vi "Progress bar DAC scan.vi"(1 "Voltage (V)":dbl format="%.3f", 2 "DAC code":u16) -> (0 "Abort":bool, 3 "Prog Bar Ref":refnum<vi>)   [LabVIEW 2015]
panel:
  in  "Abort":bool
  out "DAC code":u16(slide) scale=0.0..65535.0
  # "DAC Scan Progress"
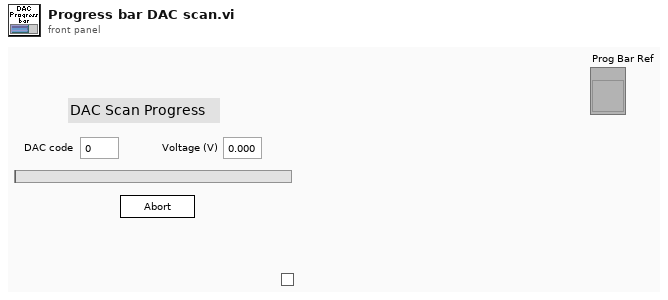
[diagram p1: front panel]
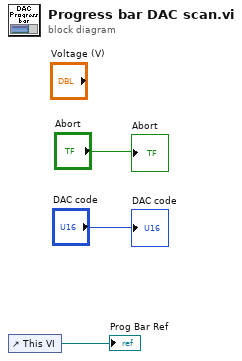
[diagram p0: block diagram]
diagram:
  n1 = control-ref of="This VI"() -> (→"Prog Bar Ref":refnum<vi>)
  "DAC code" <- "DAC code"
  "Abort" <- "Abort"
